vi "Write Configuration.vi"(8 "error in (no error)":errorcluster, 10 "Configuration":T1={"Start current"=-0.001, "End current"=0.001, "Current step"=0.0001, "Step time"=1.0} {"Step time" format="%#_6ps"; "Current step" format="%#_6pA"; "End current" format="%#_6pA"; "Start current" format="%#_6pA"}, 11 "IV in":refnum<class "IV.lvclass">) -> (0 "error out":errorcluster, 3 "IV out":refnum<class "IV.lvclass">)   [LabVIEW 2021, in "IV.lvclass"]
uses:
  IV.lvclass
  Libraries/Instruments/Controls/IV Config.ctl
  IV.lvclass/IV.ctl
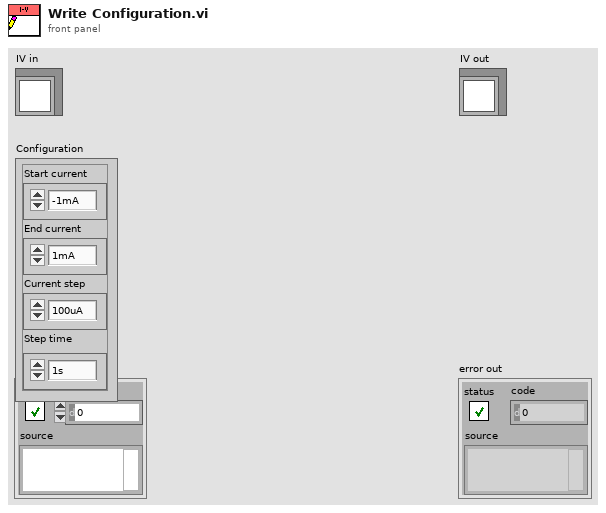
[diagram p1: front panel]
types:
  T1 = typedef "IV Config.ctl" = cluster{"Start current":dbl, "End current":dbl, "Current step":dbl, "Step time":dbl}
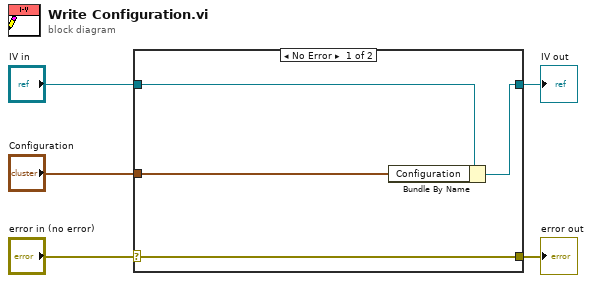
[diagram p0: block diagram]
diagram:
  n1 = case shown="No Error" "error in (no error)" {
    selector: "error in (no error)" -> [w9 w10]
    tunnel: [w9 w10] -> w4
    tunnel: [w7 w11] -> w2
    tunnel: "IV in" -> [w8 w11]
    tunnel: "Configuration" -> [w6 _]
    frame No Error {
      n2 = Bundle By Name(cluster=w8, "Configuration"=w6) -> (w7:refnum<class "IV.lvclass">)
    }
    frame Error {
    }
  }
  "error out" <- w4
  "IV out" <- w2
